vi "Check If String is Number.vi"(1 "String":string) -> (0 "Is a Number?":bool)   [LabVIEW 2020]
panel:
  # "Overview: This example checks if the string is just a number\nRequirements: LabVIEW 2012 (or compatible)\nInstructions:\n1. Insert the string to be checked\n2. Run the VI\n3. If the string is number the LED will be true"
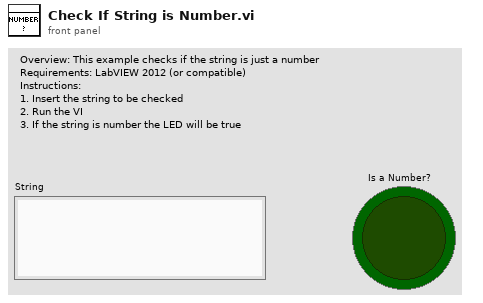
[diagram p1: front panel]
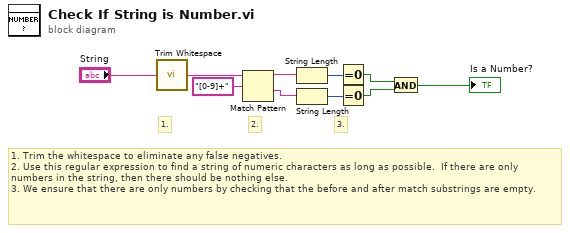
[diagram p0: block diagram]
diagram:
  # "3."
  # "2."
  # "1."
  # "1. Trim the whitespace to eliminate any false negatives.\n2. Use this regular expression to find a string of numeric characters as long as possible.  If there are only numbers in the string, then there should be nothing else.\n3. We ensure that there are only numbers by checking that the before and after match substrings are empty."
  n1 = call <vilib>:"Trim Whitespace.vi"("string"="String") -> ("trimmed string"=w1:string)  [unwired: 1 in]
  n2 = Match Pattern(string=w1, regular expression="[0-9]+") -> (before substring=w9:string, after substring=w8:string)  [unwired: 1 in, 2 out]
  n3 = String Length(string=w9) -> (length=w7:i32)
  n4 = String Length(string=w8) -> (length=w6:i32)
  n5 = Equal To 0?(x=w7) -> (x = 0?=w5:bool)
  n6 = Equal To 0?(x=w6) -> (x = 0?=w4:bool)
  n7 = And(x=w5, y=w4) -> (x .and. y?=→"Is a Number?":bool)
